vi "StartCountdown.vi"(8 "CountdownOccurrence":refnum<k4>, 9 "Teleop?":bool, 10 "CountdownStartTime":i32, 11 "Time":i32) -> ()   [LabVIEW 2015]
doc: "Starts the countdown if the current time equals the countdown start time and we're in teleop mode."
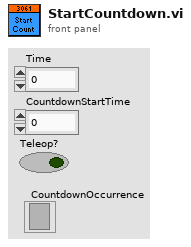
[diagram p1: front panel]
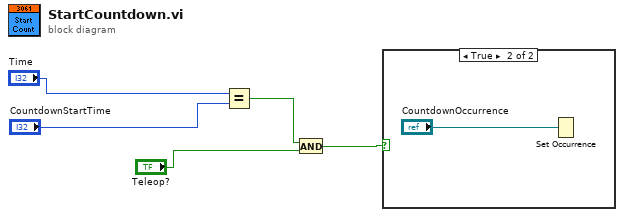
[diagram p0: block diagram]
diagram:
  n1 = Equal?(x="Time", y="CountdownStartTime") -> (x = y?=w3:bool)
  n2 = And(x=w3, y="Teleop?") -> (x .and. y?=w1:bool)
  n3 = case shown="True" w1 {
    frame False {
    }
    frame True {
      n4 = Set Occurrence("CountdownOccurrence") -> ()
    }
  }
